vi "lamp-power.vi"(8 "error in (no error)":errorcluster, 10 "Set":bool, 11 "Lamp":refnum<vi>) -> (0 "error out":errorcluster)   [LabVIEW 2016]
uses:
  controls/lamp.ctl
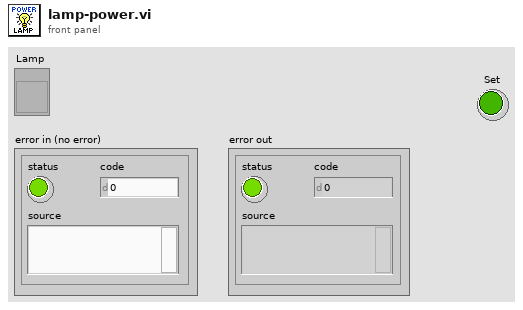
[diagram p1: front panel]
types:
  T1 = typedef "lamp.ctl" = cluster{"Port":refnum<visa-resource-name>, "Power":u16, "Is Conected?":bool, "ON":bool, "Open":bool, "Save":bool, "Model":string}
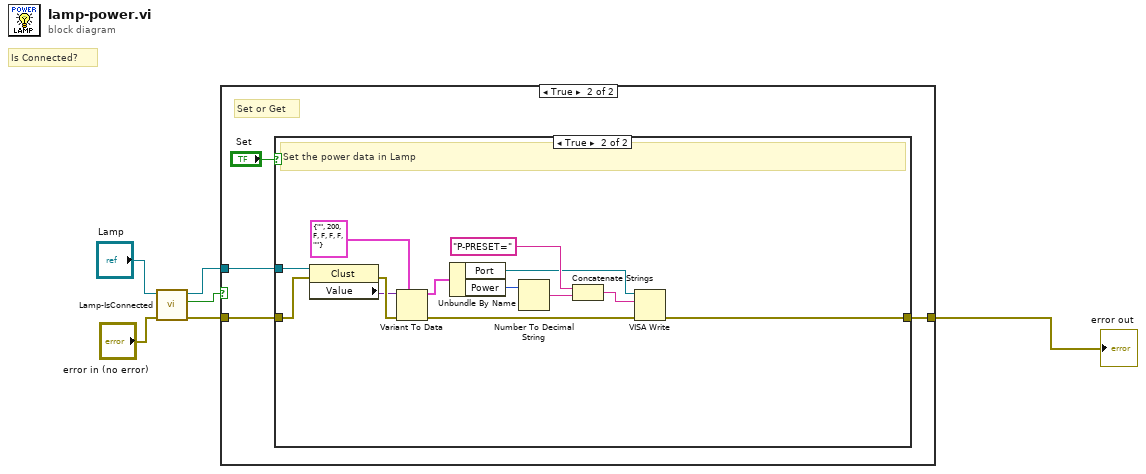
[diagram p0: block diagram]
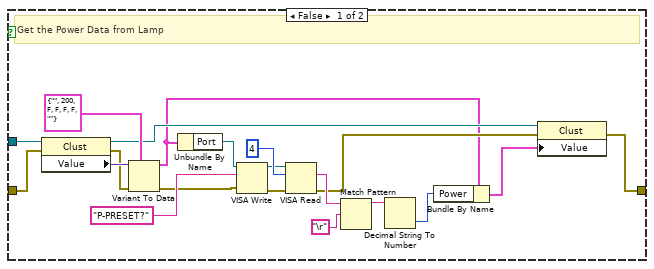
[diagram p3: hidden frame]
diagram:
  # "Is Connected?"
  n1 = call "Lamp-IsConnected.vi"("error in (no error)"="error in (no error)", "Lamp in"="Lamp") -> ("error out"=w2:errorcluster, "Connected"=w1:bool, "Lamp out"=w3:refnum<vi>)  [unwired: 7 in]
  n2 = case shown="True" w1 {
    tunnel: w2 -> [w7 w11]
    tunnel: [w7 w9] -> w6
    tunnel: w3 -> [_ w8]
    frame False {
    }
    frame True {
      # "Set or Get"
      n3 = case shown="True" "Set" {
        tunnel: [w15 w39] -> w9
        tunnel: w11 -> [w22 w37]
        tunnel: w8 -> [w23 w38]
        frame False {
          # "Get the Power Data from Lamp"
          n4 = property class="Clust"(reference=w23, error in=w22) -> (reference out=w17:refnum<vi>, error out=w20:errorcluster, "Value"=w21:variant)
          n5 = Variant To Data(error in=w20, type=T1 {"Port"="", "Power"=200, "Is Conected?"=FALSE, "ON"=FALSE, "Open"=FALSE, "Save"=FALSE, "Model"=""} ("Lamp"), Variant=w21) -> (data=w14:T1, error out=w18:errorcluster)
          n6 = Unbundle By Name(w14) -> ("Port"=w24:refnum<visa-resource-name>)
          n7 = VISA Write(VISA resource name=w24, write buffer="P-PRESET?", error in (no error)=w18) -> (VISA resource name out=w27:refnum<visa-resource-name>, error out=w26:errorcluster)  [unwired: 1 out]
          n8 = VISA Read(VISA resource name=w27, byte count=u32 4, error in (no error)=w26) -> (read buffer=w31:string, error out=w16:errorcluster)  [unwired: 2 out]
          n9 = Match Pattern(string=w31, regular expression="\r") -> (before substring=w30:string)  [unwired: 1 in, 3 out]
          n10 = Decimal String To Number(string=w30) -> (number=w12:i32)  [unwired: 2 in, 1 out]
          n11 = Bundle By Name(cluster=w14, "Power"=w12) -> (w13:T1)
          n12 = property class="Clust"(reference=w17, error in=w16, "Value"=w13) -> (error out=w15:errorcluster)  [unwired: 1 out]
        }
        frame True {
          # "Set the power data in Lamp"
          n13 = property class="Clust"(reference=w38, error in=w37) -> (error out=w35:errorcluster, "Value"=w34:variant)  [unwired: 1 out]
          n14 = Variant To Data(error in=w35, type=T1 {"Port"="", "Power"=200, "Is Conected?"=FALSE, "ON"=FALSE, "Open"=FALSE, "Save"=FALSE, "Model"=""} ("Lamp"), Variant=w34) -> (data=w33:T1, error out=w36:errorcluster)
          n15 = Unbundle By Name(w33) -> ("Port"=w40:refnum<visa-resource-name>, "Power"=w41:u16)
          n16 = Number To Decimal String(number=w41) -> (decimal integer string=w44:string)  [unwired: 1 in]
          n17 = Concatenate Strings("P-PRESET=" ("write buffer"), w44) -> (w43:string)
          n18 = VISA Write(VISA resource name=w40, write buffer=w43, error in (no error)=w36) -> (error out=w39:errorcluster)  [unwired: 2 out]
        }
      }
    }
  }
  "error out" <- w6
